vi "Measure_temp_single.vi"(6 "stop":bool, 8 "error in (no error)":errorcluster, 9 "Type # 1":i16(ring)=107 items=["B"=98, "E"=101, "J"=106, "K"=107, "N"=110, "R"=114, "S"=115, "T"=116, "Voltage"=120], 10 "Units":enum16{"C°", "F°", "K°", "R°"}(ring), 11 "IVI Refnum in":refnum<k15>) -> (0 "error out":errorcluster, 1 "handle":i16, 2 "?":dynamicdata(graph), 3 "IVI Refnum out":refnum<k15>, 5 "T2":sgl, 7 "T1":sgl)   [LabVIEW 2015]
uses:
  Program Files (x86)/Pico Technology/SDK/lib/usbtc08.dll
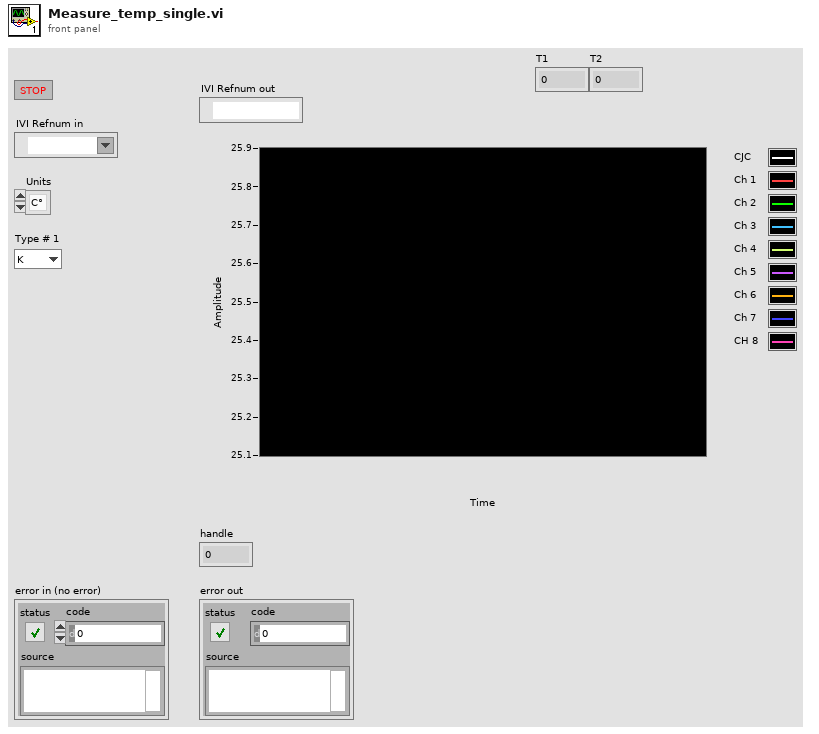
[diagram p1: front panel]
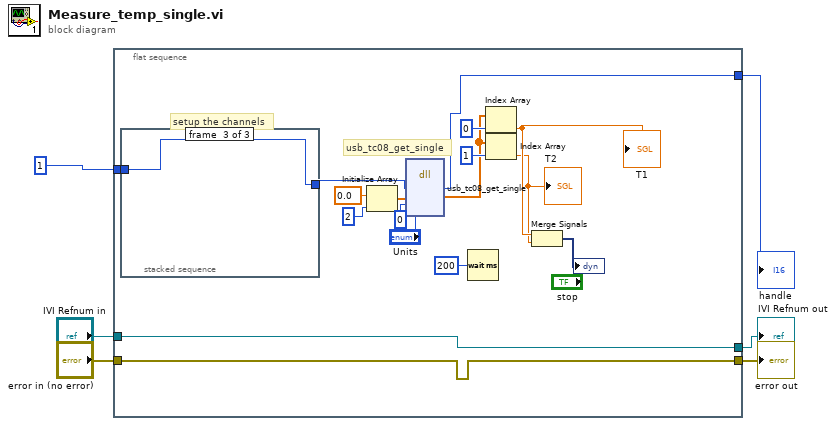
[diagram p0: block diagram]
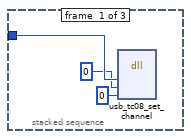
[diagram p2: hidden frame]
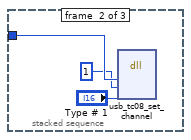
[diagram p3: hidden frame]
diagram:
  n1 = flat-sequence {
    tunnel: [w23] -> w6
    tunnel: i16 1 ("Handle 2") -> [w22]
    tunnel: [w8] -> w4
    tunnel: "IVI Refnum in" -> [w8]
    tunnel: [w7] -> w2
    tunnel: "error in (no error)" -> [w7]
    frame #0 {
      # "usb_tc08_get_single"
      # "setup the channels"
      n2 = stacked-sequence {
        tunnel: w22 -> [w26 w29 w30]
        tunnel: [_ _ w30] -> w18
        frame #0 {
          n3 = dll-call lib="C:/Program Files (x86)/Pico Technology/SDK/lib/usbtc08.dll" fn="usb_tc08_set_channel"("handle"=w26, "channel"=i16 0, "tc_type"=i8 0) -> ()  [unwired: 7 in, 2 out]
        }
        frame #1 {
          n4 = dll-call lib="C:/Program Files (x86)/Pico Technology/SDK/lib/usbtc08.dll" fn="usb_tc08_set_channel"("handle"=w29, "channel"=i16 1, "tc_type"="Type # 1") -> ()  [unwired: 7 in, 2 out]
        }
        frame #2 {
        }
      }
      n5 = Initialize Array(sgl 0.0, i16 2) -> (w21:sgl[])
      n6 = dll-call lib="C:/Program Files (x86)/Pico Technology/SDK/lib/usbtc08.dll" fn="usb_tc08_get_single"("handle"=w18, "temp_buffer"=w21, "overflow"=i16 0, "units"="Units") -> ("handle"=w23:i16, "temp_buffer"=w13:sgl[])  [unwired: 6 in, 2 out]
      n7 = Wait (ms)(milliseconds to wait=u32 200) -> ()  [unwired: 1 out]
      n8 = Index Array(array=w13, index=i16 0) -> (element=w12:sgl)
      "T1" <- w12
      n9 = Index Array(array=w13, index=i16 1) -> (element=w11:sgl)
      "T2" <- w11
      n10 = Merge Signals(w12, w11) -> (→"?":dynamicdata)
    }
  }
  "handle" <- w6
  "error out" <- w2
  "IVI Refnum out" <- w4
